vi "Transcriptor LabVIEW to VHDL code Translator Native Functions.vi"(0 "Input":variant=variant("Function Name"=variant(string "Strip Path"), "Input Datatypes"=variant(string[] ["error", "int"]), "Inputs"=variant(string[] ["error in", "x"]), "Node refnum"=variant(refnum<vi> refnum), "Output Datatypes"=variant(string[] ["int"]), "Outputs"=variant(string[] ["a"])), 11 "error in (no error)":errorcluster) -> (4 "Output":variant=variant("Defines"=variant(string[] []), "Includes"=variant(string[] []), "Replaced Code"=variant(string "/* LabVIEW system function 'Strip Path' not found. */")), 15 "error out":errorcluster)   [LabVIEW 2018]
doc: "An example of how to create the Translator to convert the LabVIEW VIs to Arduino C code."
uses:
  <vilib>/regexp/Match Regular Expression.xnode
panel:
  out "Outputs":string[](array[string])
  out "Inputs":string[](array[string])
  out "Output Datatypes":string[](array[string])
  out "Input Datatypes":string[](array[string])
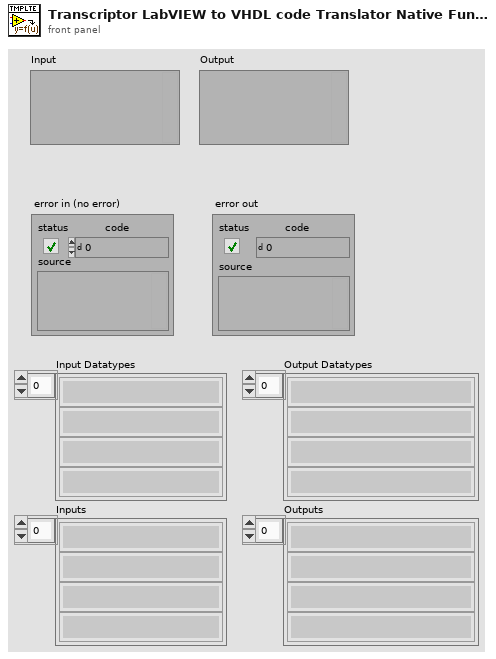
[diagram p1: front panel]
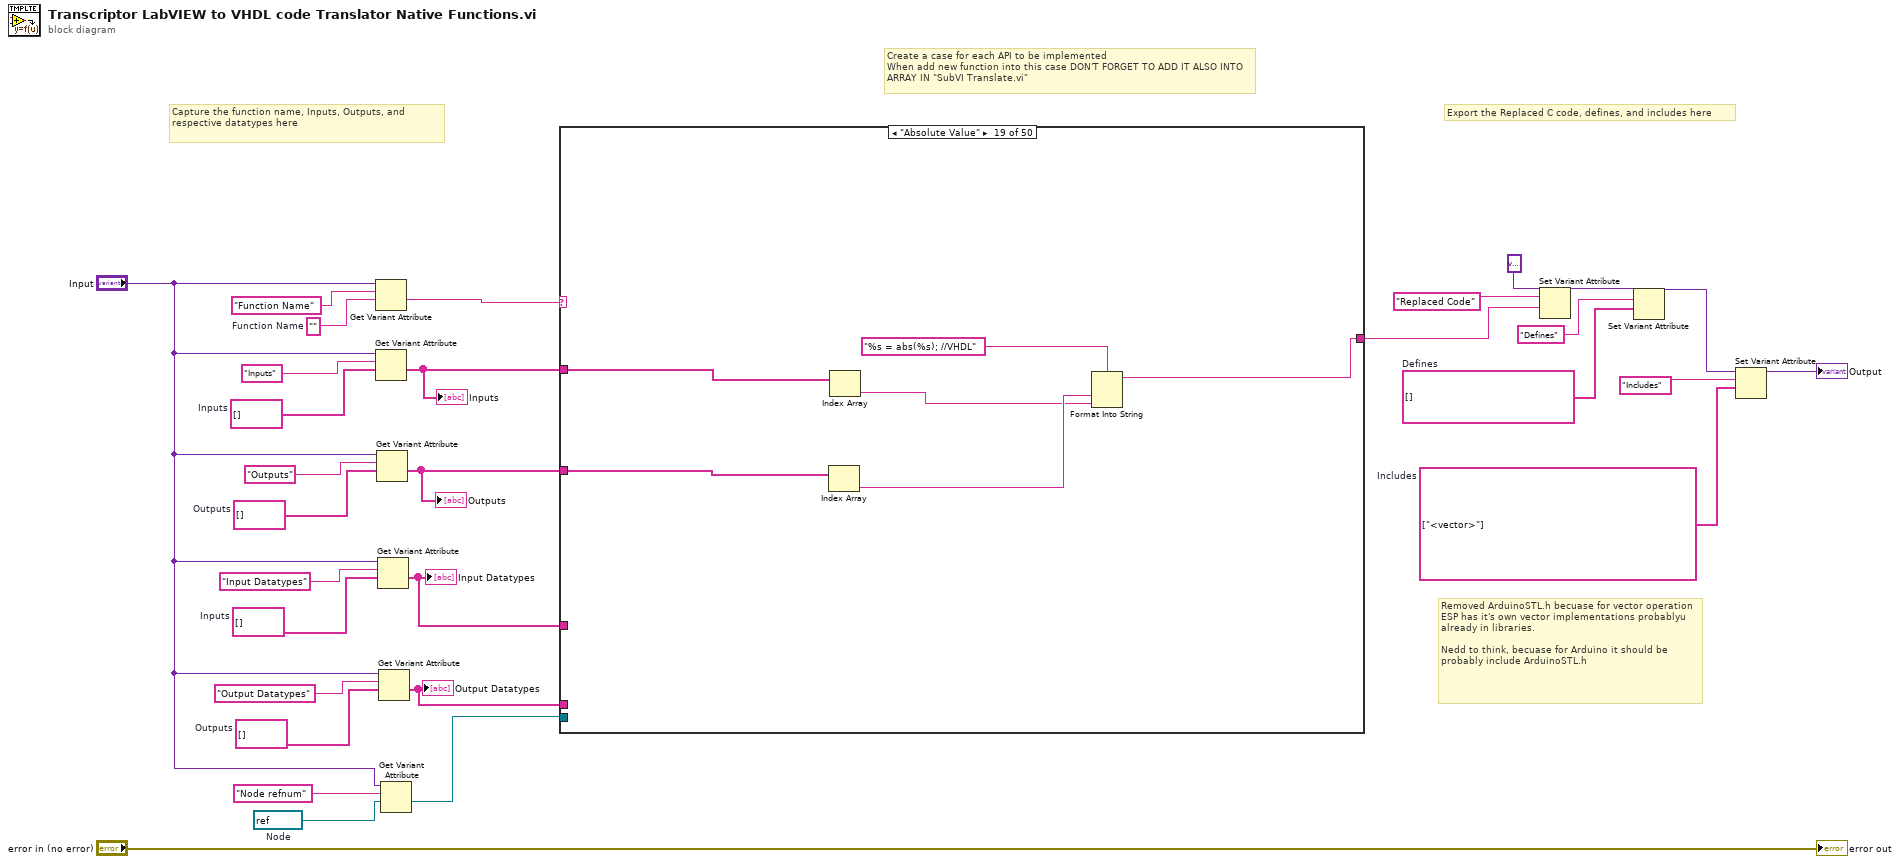
[diagram p0: block diagram]
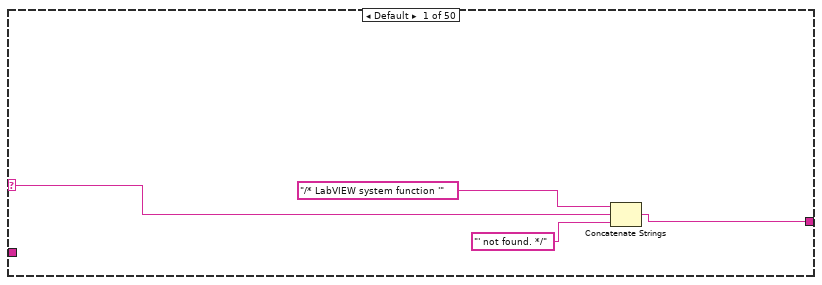
[diagram p2: hidden frame]
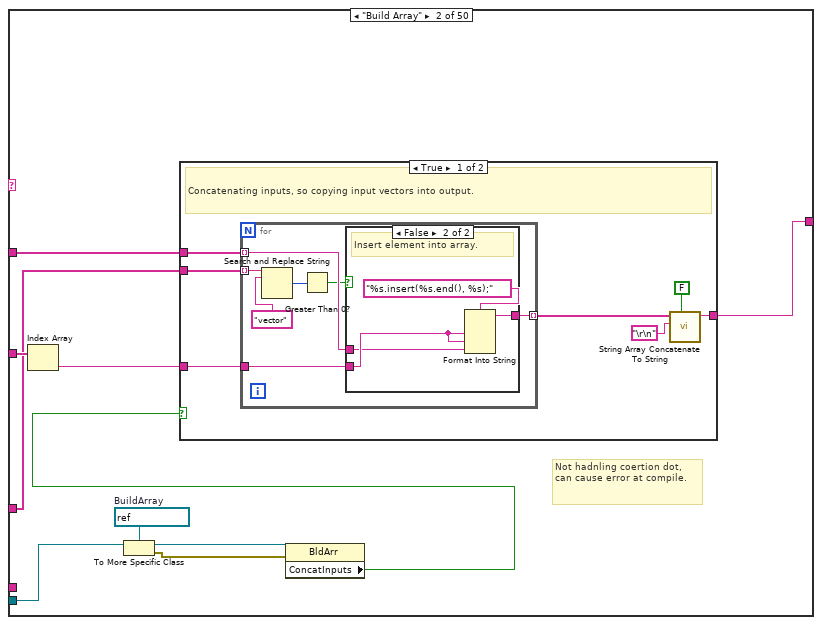
[diagram p3: hidden frame]
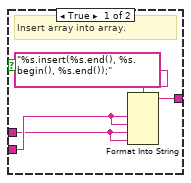
[diagram p4: hidden frame]
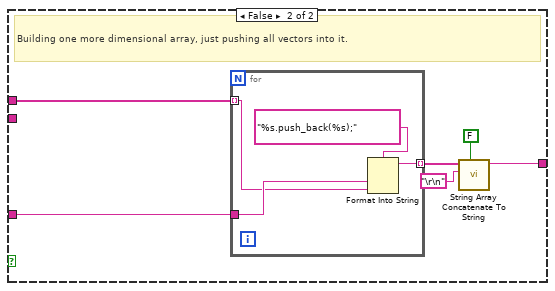
[diagram p5: hidden frame]
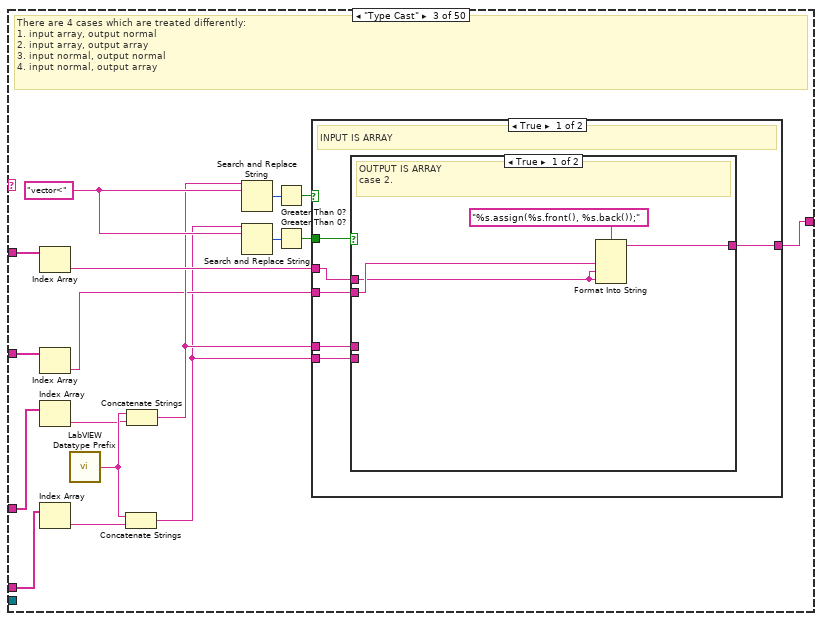
[diagram p6: hidden frame]
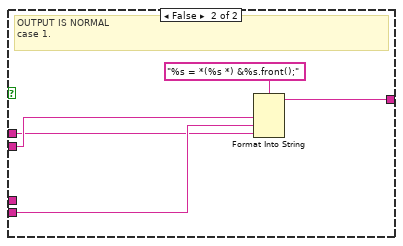
[diagram p7: hidden frame]
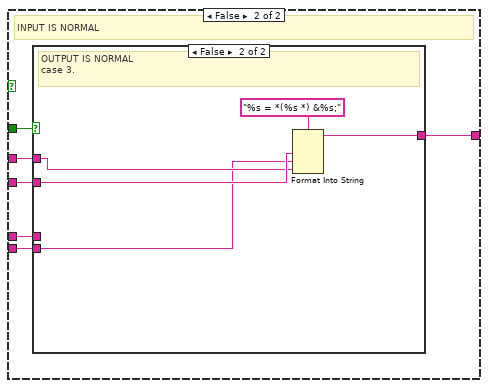
[diagram p8: hidden frame]
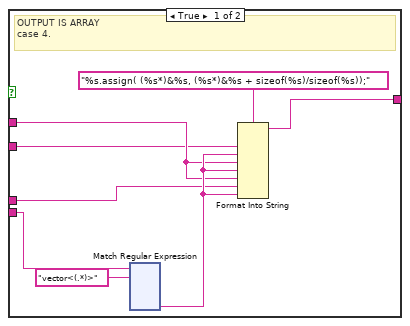
[diagram p9: hidden frame]
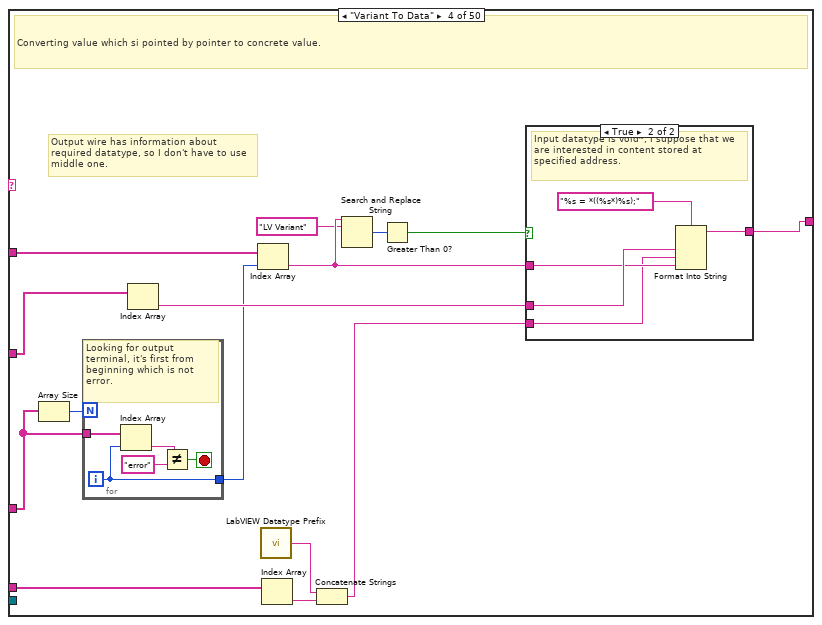
[diagram p10: hidden frame]
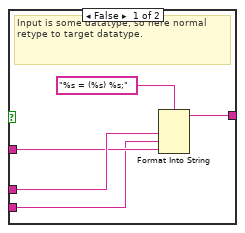
[diagram p11: hidden frame]
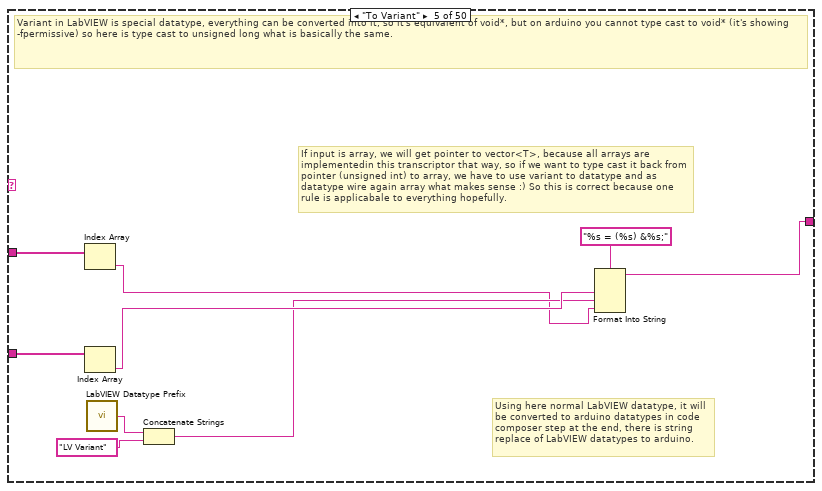
[diagram p12: hidden frame]
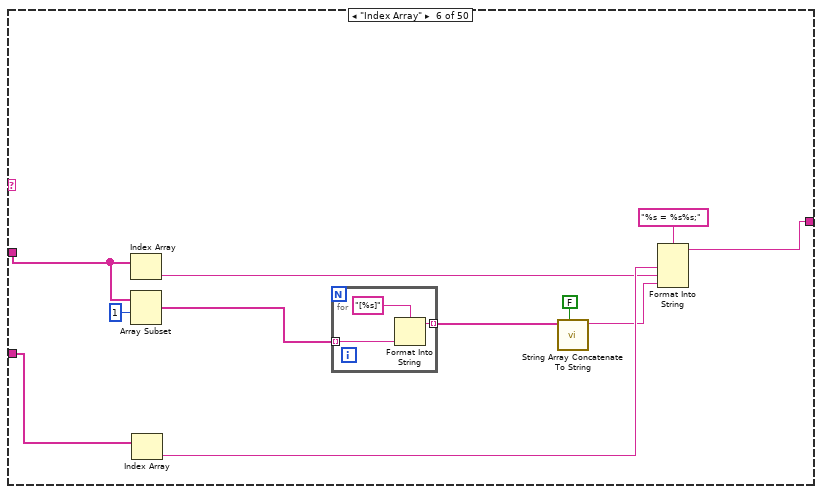
[diagram p13: hidden frame]
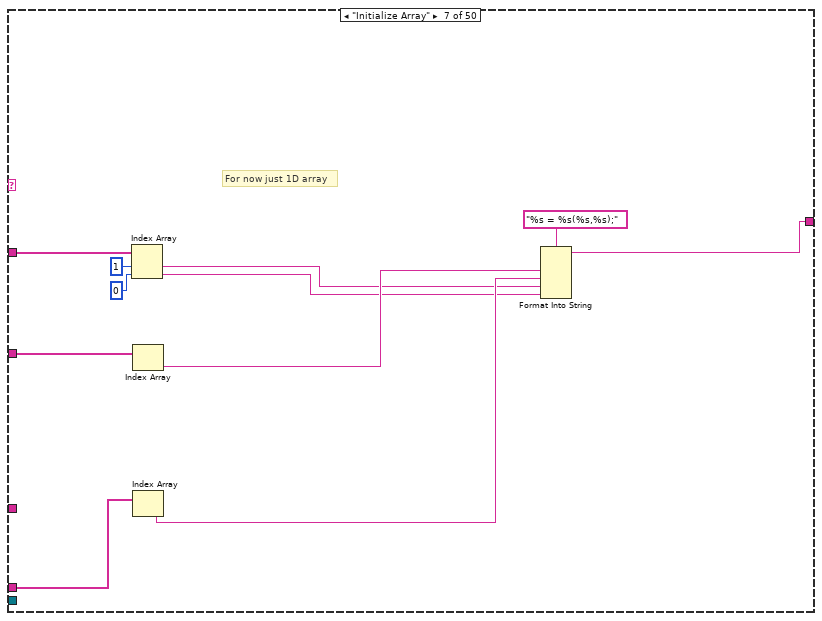
[diagram p14: hidden frame]
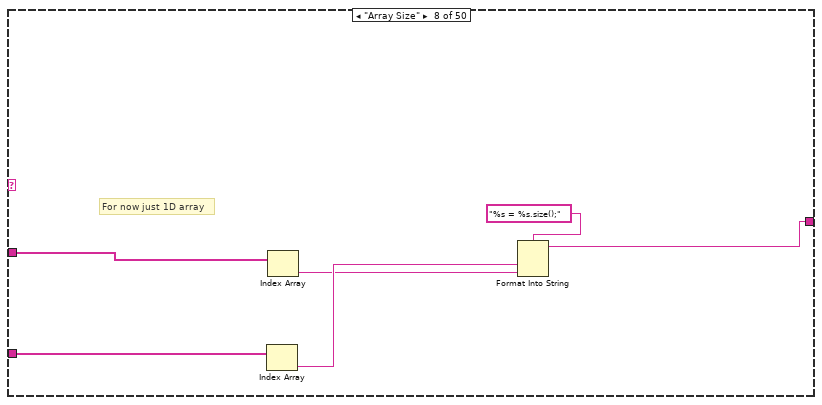
[diagram p15: hidden frame]
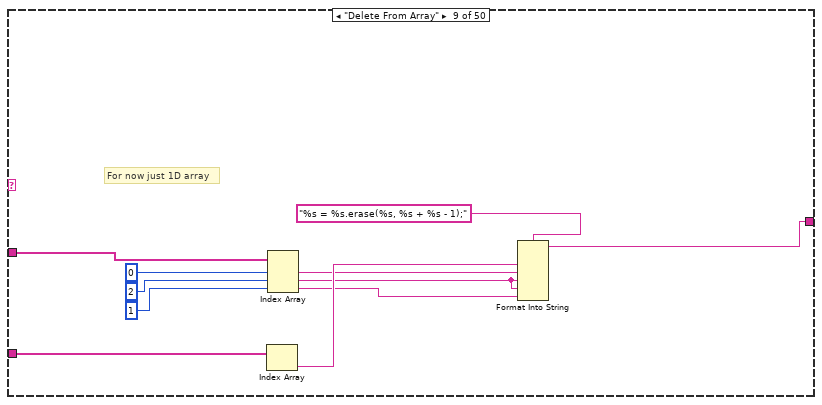
[diagram p16: hidden frame]
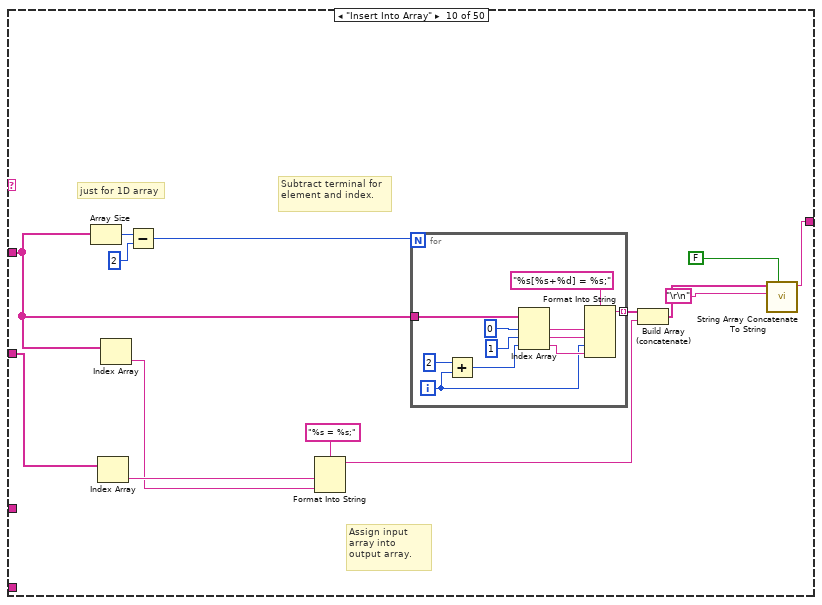
[diagram p17: hidden frame]
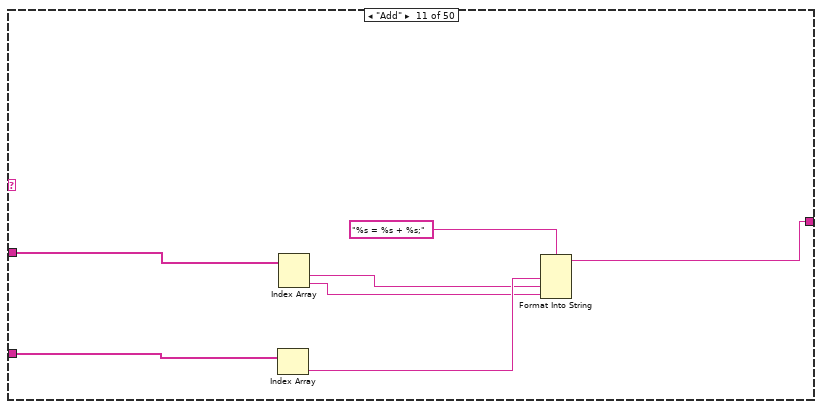
[diagram p18: hidden frame]
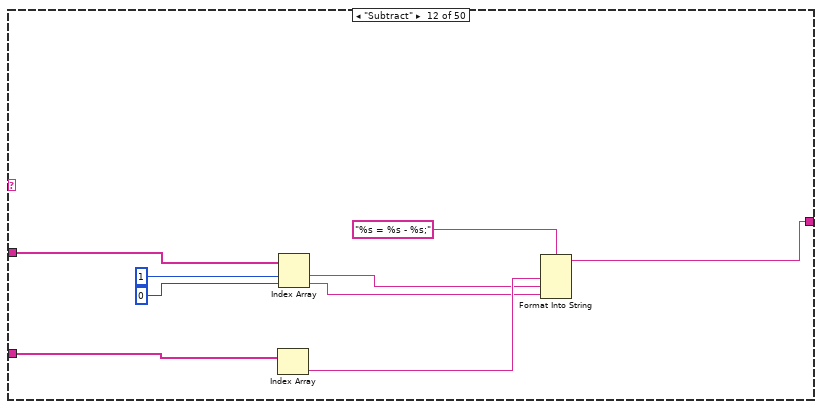
[diagram p19: hidden frame]
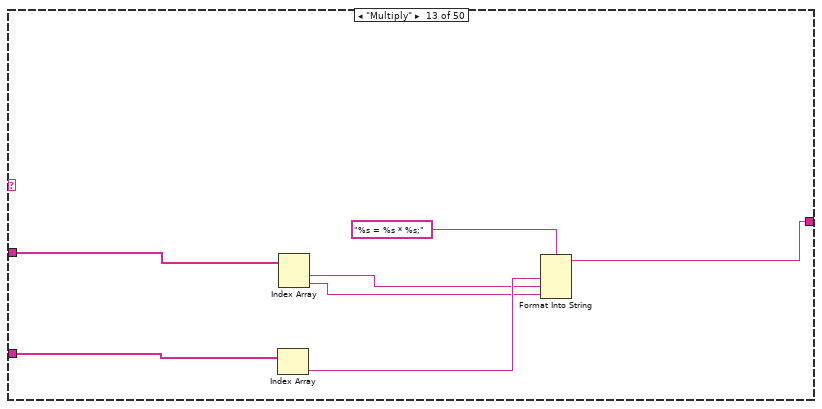
[diagram p20: hidden frame]
diagram:
  w3 = refnum<vi> refnum  # Node
  w7 = string[] []  # Defines
  w15 = string[] []  # Outputs
  w16 = string[] []  # Inputs
  w21 = string[] ["<vector>"]  # Includes
  w26 = string[] []  # Outputs
  w27 = string[] []  # Inputs
  w28 = ""  # Function Name
  # "Removed ArduinoSTL.h becuase for vector operation ESP has it's own vector implementations probablyu already in libraries.\n\nNedd to think, becuase for Arduino it should be probably include ArduinoSTL.h"
  # "Capture the function name, Inputs, Outputs, and respective datatypes here"
  # "Export the Replaced C code, defines, and includes here"
  # "Create a case for each API to be implemented\nWhen add new function into this case DON'T FORGET TO ADD IT ALSO INTO ARRAY IN \"SubVI Translate.vi\""
  n1 = Get Variant Attribute(Variant="Input", name="Function Name", default value (empty Variant)=w28) -> (value=w23:string)  [unwired: 1 in, 3 out]
  n2 = Get Variant Attribute(Variant="Input", name="Inputs", default value (empty Variant)=w27) -> (value=w12:string[])  [unwired: 1 in, 3 out]
  "Inputs" <- w12
  n3 = Get Variant Attribute(Variant="Input", name="Outputs", default value (empty Variant)=w26) -> (value=w13:string[])  [unwired: 1 in, 3 out]
  "Outputs" <- w13
  n4 = Get Variant Attribute(Variant="Input", name="Input Datatypes", default value (empty Variant)=w16) -> (value=w6:string[])  [unwired: 1 in, 3 out]
  "Input Datatypes" <- w6
  n5 = Get Variant Attribute(Variant="Input", name="Output Datatypes", default value (empty Variant)=w15) -> (value=w1:string[])  [unwired: 1 in, 3 out]
  "Output Datatypes" <- w1
  n6 = Get Variant Attribute(Variant="Input", name="Node refnum", default value (empty Variant)=w3) -> (value=w2:refnum<vi>)  [unwired: 1 in, 3 out]
  n7 = case shown="\"Absolute Value\"" w23 {
    selector: w23 -> [w33 _ _ _ _ _ _ _ _ _ _ _ _ _ _ _ _ _ _ _ _ _ _ _ _ _ _ _ _ _ _ _ _ _ _ _ _ _ _ _ _ _ _ _ _ _ _ _ _ _]
    tunnel: [w31 w41 w93 w258 w282 w289 w297 w308 w319 w336 w350 w359 w366 w375 w382 w391 w400 w407 w413 w419 w425 w431 w437 w443 w449 w455 w466 w477 w483 w490 w496 w503 w515 w521 w525 w532 w537 w552 w569 w579 w589 w599 w605 w611 w617 w623 w629 w635 w641 w647] -> w22
    tunnel: w12 -> [_ w43 w92 w251 w281 w288 w307 w313 w324 w329 w356 w365 w372 w381 w388 w397 w406 w412 w418 w424 w430 w436 w442 w448 w454 w460 w465 w474 w489 w495 w502 w509 w512 w524 w528 w534 w536 w554 w566 w576 w586 w598 w604 w610 w616 w622 w628 w634 w640 w646]
    tunnel: w13 -> [_ w44 w91 w257 w280 w293 w306 w311 w322 w332 w354 w363 w370 w379 w386 w395 w404 w410 w416 w422 w428 w434 w440 w446 w452 w458 w470 w481 w487 w493 w500 w507 w519 _ _ w530 w535 w553 w563 w573 w583 w594 w603 w609 w615 w621 w627 w633 w639 w645]
    tunnel: w6 -> [_ w35 w83 w249 _ _ _ _ _ _ _ _ _ _ _ _ _ _ _ _ _ _ _ _ _ _ _ _ _ _ _ _ _ _ _ _ _ _ _ _ _ _ _ _ _ _ _ _ _ _]
    tunnel: w2 -> [_ w40 _ _ _ _ _ _ _ _ _ _ _ _ _ _ _ _ _ _ _ _ _ _ _ _ _ _ _ _ _ _ _ _ _ _ _ _ _ _ _ _ _ _ _ _ _ _ _ _]
    tunnel: w1 -> [_ _ w89 w252 _ _ w302 _ _ _ _ _ _ _ _ _ _ _ _ _ _ _ _ _ _ _ _ _ _ _ _ _ _ _ _ _ _ _ _ _ _ _ _ _ _ _ _ _ _ _]
    frame Default {
      n8 = Concatenate Strings("/* LabVIEW system function '", w33, "' not found. */") -> (w31:string)
    }
    frame "Build Array" {
      w39 = refnum<vi> refnum  # BuildArray
      # "Not hadnling coertion dot, can cause error at compile."
      n9 = Index Array(array=w44) -> (element=w42:string)  [unwired: 1 in]
      n10 = To More Specific Class(target class=w39, reference=w40) -> (specific class reference=w38:refnum<vi>, error out=w37:errorcluster)  [unwired: 1 in]
      n11 = property class="BldArr"(reference=w38, error in=w37) -> ("ConcatInputs"=w36:bool)  [unwired: 2 out]
      n12 = case shown="True" w36 {
        tunnel: w43 -> [w51 w72]
        tunnel: w42 -> [w50 w71]
        tunnel: [w46 w67] -> w41
        tunnel: w35 -> [w45 _]
        frame True {
          # "Concatenating inputs, so copying input vectors into output."
          n13 = for {
            tunnel: w51 -> [w57] mode=indexing
            tunnel: w50 -> [w58]
            tunnel: [w56] -> w49 mode=indexing
            tunnel: w45 -> [w55] mode=indexing
            n14 = Search and Replace String(input string=w55, search string="vector" ("name")) -> (number of replacements=w53:i32)  [unwired: 6 in, 3 out]
            n15 = Greater Than 0?(x=w53) -> (x > 0?=w52:bool)
            n16 = case shown="False" w52 {
              tunnel: w58 -> [w61 w65]
              tunnel: w57 -> [w60 w64]
              tunnel: [w59 w63] -> w56
              frame True {
                # "Insert array into array."
                n17 = Format Into String(format string="%s.insert(%s.end(), %s.begin(), %s.end());" ("name"), w61, w61, w60, w60) -> (resulting string=w59:string)  [unwired: 2 in, 1 out]
              }
              frame False {
                # "Insert element into array."
                n18 = Format Into String(format string="%s.insert(%s.end(), %s);" ("name"), w65, w65, w64) -> (resulting string=w63:string)  [unwired: 2 in, 1 out]
              }
            }
          }
          n19 = call "String Array Concatenate To String.vi"("insert last delimiter?"=FALSE, "Delimiter char"="\r\n", "Array String In"=w49) -> ("String"=w46:string)  [unwired: 8 in]
        }
        frame False {
          # "Building one more dimensional array, just pushing all vectors into it."
          n20 = for {
            tunnel: w72 -> [w74] mode=indexing
            tunnel: w71 -> [w75]
            tunnel: [w73] -> w70 mode=indexing
            n21 = Format Into String(format string="%s.push_back(%s);" ("name"), w75, w74) -> (resulting string=w73:string)  [unwired: 2 in, 1 out]
          }
          n22 = call "String Array Concatenate To String.vi"("insert last delimiter?"=FALSE, "Delimiter char"="\r\n", "Array String In"=w70) -> ("String"=w67:string)  [unwired: 8 in]
        }
      }
    }
    frame "Type Cast" {
      w86 = "vector<" ("search string")
      # "There are 4 cases which are treated differently:\n1. input array, output normal\n2. input array, output array\n3. input normal, output normal\n4. input normal, output array"
      n23 = Index Array(array=w92) -> (element=w82:string)  [unwired: 1 in]
      n24 = Index Array(array=w91) -> (element=w78:string)  [unwired: 1 in]
      n25 = Index Array(array=w83) -> (element=w80:string)  [unwired: 1 in]
      n26 = Index Array(array=w89) -> (element=w90:string)  [unwired: 1 in]
      n27 = call "LabVIEW Datatype Prefix.vi"() -> ("datatype prefix"=w81:string)
      n28 = Concatenate Strings(w81, w90) -> (w77:string)
      n29 = Concatenate Strings(w81, w80) -> (w79:string)
      n30 = Search and Replace String(input string=w79, search string=w86) -> (number of replacements=w88:i32)  [unwired: 6 in, 3 out]
      n31 = Search and Replace String(input string=w77, search string=w86) -> (number of replacements=w87:i32)  [unwired: 6 in, 3 out]
      n32 = Greater Than 0?(x=w88) -> (x > 0?=w85:bool)
      n33 = Greater Than 0?(x=w87) -> (x > 0?=w84:bool)
      n34 = case shown="True" w85 {
        tunnel: [w99 w114] -> w93
        tunnel: w82 -> [w98 w113]
        tunnel: w78 -> [w97 w112]
        tunnel: w84 -> [w96 w111]
        tunnel: w79 -> [w95 w110]
        tunnel: w77 -> [w94 w109]
        frame True {
          # "INPUT IS ARRAY"
          n35 = case shown="True" w96 {
            tunnel: [w102 w107] -> w99
            tunnel: w97 -> [w101 w106]
            tunnel: w98 -> [w100 w104]
            tunnel: w95 -> [_ _]
            tunnel: w94 -> [_ w105]
            frame True {
              # "OUTPUT IS ARRAY\ncase 2."
              n36 = Format Into String(format string="%s.assign(%s.front(), %s.back());" ("name"), w101, w100, w100) -> (resulting string=w102:string)  [unwired: 2 in, 1 out]
            }
            frame False {
              # "OUTPUT IS NORMAL\ncase 1."
              n37 = Format Into String(format string="%s = *(%s *) &%s.front();" ("name"), w106, w105, w104) -> (resulting string=w107:string)  [unwired: 2 in, 1 out]
            }
          }
        }
        frame False {
          # "INPUT IS NORMAL"
          n38 = case shown="False" w111 {
            tunnel: [w119 w242] -> w114
            tunnel: w112 -> [w117 w241]
            tunnel: w113 -> [w118 w240]
            tunnel: w110 -> [w116 _]
            tunnel: w109 -> [w115 w239]
            frame True {
              # "OUTPUT IS ARRAY\ncase 4."
              n39 = xnode "Match Regular Expression"("input string"=w115, "regular expression"="vector<(.*)>") -> ("submatch 1"=w120:string)  [unwired: 4 in, 5 out]
              n40 = Format Into String(format string="%s.assign( (%s*)&%s, (%s*)&%s + sizeof(%s)/sizeof(%s));" ("name"), w117, w120, w118, w120, w118, w116, w120) -> (resulting string=w119:string)  [unwired: 2 in, 1 out]
            }
            frame False {
              # "OUTPUT IS NORMAL\ncase 3."
              n41 = Format Into String(format string="%s = *(%s *) &%s;" ("name"), w241, w239, w240) -> (resulting string=w242:string)  [unwired: 2 in, 1 out]
            }
          }
        }
      }
    }
    frame "Variant To Data" {
      # "Output wire has information about required datatype, so I don't have to use middle one."
      # "Converting value which si pointed by pointer to concrete value."
      n42 = Array Size(array=w249) -> (size(s)=w250:i32)
      n43 = for {
        N: w250 -> [_]
        tunnel: w249 -> [w273]
        tunnel: [w269] -> w248
        i -> [w269]
        stop <- w272 stop-if-true
        # "Looking for output terminal, it's first from beginning which is not error."
        n44 = Index Array(array=w273, index=w269) -> (element=w271:string)
        n45 = Not Equal?(x=w271, y="error") -> (x != y?=w272:bool)
      }
      n46 = Index Array(array=w257) -> (element=w256:string)  [unwired: 1 in]
      n47 = Index Array(array=w251, index=w248) -> (element=w247:string)
      n48 = call "LabVIEW Datatype Prefix.vi"() -> ("datatype prefix"=w253:string)
      n49 = Index Array(array=w252) -> (element=w255:string)  [unwired: 1 in]
      n50 = Concatenate Strings(w253, w255) -> (w254:string)
      n51 = Search and Replace String(input string=w247, search string="LV Variant") -> (number of replacements=w245:i32)  [unwired: 6 in, 3 out]
      n52 = Greater Than 0?(x=w245) -> (x > 0?=w244:bool)
      n53 = case shown="True" w244 {
        tunnel: [w262 w267] -> w258
        tunnel: w256 -> [w261 w266]
        tunnel: w247 -> [w260 w265]
        tunnel: w254 -> [w259 w264]
        frame False {
          # "Input is some datatype, so here normal retype to target datatype."
          n54 = Format Into String(format string="%s = (%s) %s;" ("name"), w261, w259, w260) -> (resulting string=w262:string)  [unwired: 2 in, 1 out]
        }
        frame True {
          # "Input datatype is void*, I suppose that we are interested in content stored at specified address."
          n55 = Format Into String(format string="%s = *((%s*)%s);" ("name"), w266, w264, w265) -> (resulting string=w267:string)  [unwired: 2 in, 1 out]
        }
      }
    }
    frame "To Variant" {
      # "If input is array, we will get pointer to vector<T>, because all arrays are implementedin this transcriptor that way, so if we want to type cast it back from pointer (unsigned int) to array, we have to use variant to datatype and as datatype wire again array what makes sense :) So this is correct because one rule is applicabale to everything hopefully."
      # "Using here normal LabVIEW datatype, it will be converted to arduino datatypes in code composer step at the end, there is string replace of LabVIEW datatypes to arduino."
      # "Variant in LabVIEW is special datatype, everything can be converted into it, so it's equivalent of void*, but on arduino you cannot type cast to void* (it's showing -fpermissive) so here is type cast to unsigned long what is basically the same."
      n56 = Index Array(array=w281) -> (element=w275:string)  [unwired: 1 in]
      n57 = Index Array(array=w280) -> (element=w279:string)  [unwired: 1 in]
      n58 = call "LabVIEW Datatype Prefix.vi"() -> ("datatype prefix"=w278:string)
      n59 = Concatenate Strings(w278, "LV Variant" ("string")) -> (w276:string)
      n60 = Format Into String(format string="%s = (%s) &%s;", w279, w276, w275) -> (resulting string=w282:string)  [unwired: 2 in, 1 out]
    }
    frame "Index Array" {
      n61 = Index Array(array=w288) -> (element=w290:string)  [unwired: 1 in]
      n62 = Array Subset(array=w288, index=1) -> (w286:string[])  [unwired: 1 in]
      n63 = Index Array(array=w293) -> (element=w291:string)  [unwired: 1 in]
      n64 = for {
        tunnel: w286 -> [w295] mode=indexing
        tunnel: [w294] -> w284 mode=indexing
        n65 = Format Into String(format string="[%s]", w295) -> (resulting string=w294:string)  [unwired: 2 in, 1 out]
      }
      n66 = call "String Array Concatenate To String.vi"("insert last delimiter?"=FALSE, "Array String In"=w284) -> ("String"=w283:string)  [unwired: 9 in]
      n67 = Format Into String(format string="%s = %s%s;", w291, w290, w283) -> (resulting string=w289:string)  [unwired: 2 in, 1 out]
    }
    frame "Initialize Array" {
      # "For now just 1D array"
      n68 = Index Array(array=w307, index #1=1 ("index"), index #2=0 ("index")) -> (element #1=w299:string, element #2=w298:string)
      n69 = Index Array(array=w306) -> (element=w304:string)  [unwired: 1 in]
      n70 = Index Array(array=w302) -> (element=w303:string)  [unwired: 1 in]
      n71 = Format Into String(format string="%s = %s(%s,%s);", w304, w303, w299, w298) -> (resulting string=w297:string)  [unwired: 2 in, 1 out]
    }
    frame "Array Size" {
      # "For now just 1D array"
      n72 = Index Array(array=w311) -> (element=w310:string)  [unwired: 1 in]
      n73 = Index Array(array=w313) -> (element=w309:string)  [unwired: 1 in]
      n74 = Format Into String(format string="%s = %s.size();", w310, w309) -> (resulting string=w308:string)  [unwired: 2 in, 1 out]
    }
    frame "Delete From Array" {
      # "For now just 1D array"
      n75 = Index Array(array=w322) -> (element=w321:string)  [unwired: 1 in]
      n76 = Index Array(array=w324, index #1=0 ("index"), index #2=2 ("index"), index #3=1 ("index")) -> (element #1=w320:string, element #2=w315:string, element #3=w314:string)
      n77 = Format Into String(format string="%s = %s.erase(%s, %s + %s - 1);", w321, w320, w315, w315, w314) -> (resulting string=w319:string)  [unwired: 2 in, 1 out]
    }
    frame "Insert Into Array" {
      # "just for 1D array"
      # "Subtract terminal for element and index."
      # "Assign input array into output array."
      n78 = Array Size(array=w329) -> (size(s)=w334:i32)
      n79 = Index Array(array=w332) -> (element=w330:string)  [unwired: 1 in]
      n80 = Index Array(array=w329) -> (element=w328:string)  [unwired: 1 in]
      n81 = Subtract(x=w334, y=2) -> (x-y=w335:i32)
      n82 = Format Into String(format string="%s = %s;", w330, w328) -> (resulting string=w326:string)  [unwired: 2 in, 1 out]
      n83 = for {
        N: w335 -> [_]
        tunnel: w329 -> [w346]
        tunnel: [w347] -> w327 mode=indexing
        i -> [w342]
        n84 = Add(x=2, y=w342) -> (x+y=w341:i32)
        n85 = Index Array(array=w346, index #1=0 ("index"), index #2=1 ("index"), index #3=w341) -> (element #1=w339:string, element #2=w348:string, element #3=w344:string)
        n86 = Format Into String(format string="%s[%s+%d] = %s;", w339, w348, w342, w344) -> (resulting string=w347:string)  [unwired: 2 in, 1 out]
      }
      n87 = Build Array (concatenate)(w327, w326) -> (w325:string[])
      n88 = call "String Array Concatenate To String.vi"("insert last delimiter?"=FALSE, "Delimiter char"="\r\n", "Array String In"=w325) -> ("String"=w336:string)  [unwired: 8 in]
    }
    frame "Add" {
      n89 = Index Array(array=w354) -> (element=w353:string)  [unwired: 1 in]
      n90 = Index Array(array=w356) -> (element #1=w352:string, element #2=w351:string)  [unwired: 2 in]
      n91 = Format Into String(format string="%s = %s + %s;", w353, w352, w351) -> (resulting string=w350:string)  [unwired: 2 in, 1 out]
    }
    frame "Subtract" {
      n92 = Index Array(array=w363) -> (element=w362:string)  [unwired: 1 in]
      n93 = Index Array(array=w365, index #1=1 ("index"), index #2=0 ("index")) -> (element #1=w361:string, element #2=w360:string)
      n94 = Format Into String(format string="%s = %s - %s;", w362, w361, w360) -> (resulting string=w359:string)  [unwired: 2 in, 1 out]
    }
    frame "Multiply" {
      n95 = Index Array(array=w370) -> (element=w369:string)  [unwired: 1 in]
      n96 = Index Array(array=w372) -> (element #1=w368:string, element #2=w367:string)  [unwired: 2 in]
      n97 = Format Into String(format string="%s = %s * %s;", w369, w368, w367) -> (resulting string=w366:string)  [unwired: 2 in, 1 out]
    }
    frame "Divide" {
      n98 = Index Array(array=w379) -> (element=w378:string)  [unwired: 1 in]
      n99 = Index Array(array=w381, index #1=1 ("index"), index #2=0 ("index")) -> (element #1=w377:string, element #2=w376:string)
      n100 = Format Into String(format string="%s = %s / %s;", w378, w377, w376) -> (resulting string=w375:string)  [unwired: 2 in, 1 out]
    }
    frame "Equal?" {
      n101 = Index Array(array=w386) -> (element=w385:string)  [unwired: 1 in]
      n102 = Index Array(array=w388) -> (element #1=w384:string, element #2=w383:string)  [unwired: 2 in]
      n103 = Format Into String(format string="%s = %s == %s;", w385, w384, w383) -> (resulting string=w382:string)  [unwired: 2 in, 1 out]
    }
    frame "Less?" {
      n104 = Index Array(array=w395) -> (element=w394:string)  [unwired: 1 in]
      n105 = Index Array(array=w397, index #1=1 ("index"), index #2=0 ("index")) -> (element #1=w393:string, element #2=w392:string)
      n106 = Format Into String(format string="%s = %s < %s;", w394, w393, w392) -> (resulting string=w391:string)  [unwired: 2 in, 1 out]
    }
    frame "Greater?" {
      n107 = Index Array(array=w404) -> (element=w403:string)  [unwired: 1 in]
      n108 = Index Array(array=w406, index #1=1 ("index"), index #2=0 ("index")) -> (element #1=w402:string, element #2=w401:string)
      n109 = Format Into String(format string="%s = %s > %s;", w403, w402, w401) -> (resulting string=w400:string)  [unwired: 2 in, 1 out]
    }
    frame "Not" {
      n110 = Index Array(array=w410) -> (element=w409:string)  [unwired: 1 in]
      n111 = Index Array(array=w412) -> (element=w408:string)  [unwired: 1 in]
      n112 = Format Into String(format string="%s = !%s;", w409, w408) -> (resulting string=w407:string)  [unwired: 2 in, 1 out]
    }
    frame "Absolute Value" {
      n113 = Index Array(array=w416) -> (element=w415:string)  [unwired: 1 in]
      n114 = Index Array(array=w418) -> (element=w414:string)  [unwired: 1 in]
      n115 = Format Into String(format string="%s = abs(%s); //VHDL", w415, w414) -> (resulting string=w413:string)  [unwired: 2 in, 1 out]
    }
    frame "Increment" {
      n116 = Index Array(array=w422) -> (element=w421:string)  [unwired: 1 in]
      n117 = Index Array(array=w424) -> (element=w420:string)  [unwired: 1 in]
      n118 = Format Into String(format string="%s = %s + 1;", w421, w420) -> (resulting string=w419:string)  [unwired: 2 in, 1 out]
    }
    frame "Decrement" {
      n119 = Index Array(array=w428) -> (element=w427:string)  [unwired: 1 in]
      n120 = Index Array(array=w430) -> (element=w426:string)  [unwired: 1 in]
      n121 = Format Into String(format string="%s = %s - 1;", w427, w426) -> (resulting string=w425:string)  [unwired: 2 in, 1 out]
    }
    frame "Equal To 0?" {
      n122 = Index Array(array=w434) -> (element=w433:string)  [unwired: 1 in]
      n123 = Index Array(array=w436) -> (element=w432:string)  [unwired: 1 in]
      n124 = Format Into String(format string="%s = (%s == 0);", w433, w432) -> (resulting string=w431:string)  [unwired: 2 in, 1 out]
    }
    frame "Greater Than 0?" {
      n125 = Index Array(array=w440) -> (element=w439:string)  [unwired: 1 in]
      n126 = Index Array(array=w442) -> (element=w438:string)  [unwired: 1 in]
      n127 = Format Into String(format string="%s = (%s > 0);", w439, w438) -> (resulting string=w437:string)  [unwired: 2 in, 1 out]
    }
    frame "Less Than 0?" {
      n128 = Index Array(array=w446) -> (element=w445:string)  [unwired: 1 in]
      n129 = Index Array(array=w448) -> (element=w444:string)  [unwired: 1 in]
      n130 = Format Into String(format string="%s = (%s < 0);", w445, w444) -> (resulting string=w443:string)  [unwired: 2 in, 1 out]
    }
    frame "Greater Or Equal To 0?" {
      n131 = Index Array(array=w452) -> (element=w451:string)  [unwired: 1 in]
      n132 = Index Array(array=w454) -> (element=w450:string)  [unwired: 1 in]
      n133 = Format Into String(format string="%s = (%s >= 0);", w451, w450) -> (resulting string=w449:string)  [unwired: 2 in, 1 out]
    }
    frame "Less Or Equal To 0?" {
      n134 = Index Array(array=w458) -> (element=w457:string)  [unwired: 1 in]
      n135 = Index Array(array=w460) -> (element=w456:string)  [unwired: 1 in]
      n136 = Format Into String(format string="%s = (%s <= 0);", w457, w456) -> (resulting string=w455:string)  [unwired: 2 in, 1 out]
    }
    frame "Greater Or Equal?" {
      n137 = Array Size(array=w465) -> (size(s)=w463:i32)
      n138 = Decrement(x=w463) -> (x-1=w461:i32)
      n139 = Decrement(x=w463) -> (x-1=w464:i32)
      n140 = Decrement(x=w461) -> (x-1=w462:i32)
      n141 = Index Array(array=w470) -> (element=w469:string)  [unwired: 1 in]
      n142 = Index Array(array=w465, index #1=w464, index #2=w462) -> (element #1=w468:string, element #2=w467:string)
      n143 = Format Into String(format string="%s = (%s >= %s);", w469, w468, w467) -> (resulting string=w466:string)  [unwired: 2 in, 1 out]
    }
    frame "Less Or Equal?" {
      n144 = Array Size(array=w474) -> (size(s)=w476:i32)
      n145 = Decrement(x=w476) -> (x-1=w475:i32)
      n146 = Decrement(x=w476) -> (x-1=w473:i32)
      n147 = Decrement(x=w475) -> (x-1=w472:i32)
      n148 = Index Array(array=w481) -> (element=w480:string)  [unwired: 1 in]
      n149 = Index Array(array=w474, index #1=w473, index #2=w472) -> (element #1=w479:string, element #2=w478:string)
      n150 = Format Into String(format string="%s = (%s <= %s);", w480, w479, w478) -> (resulting string=w477:string)  [unwired: 2 in, 1 out]
    }
    frame "Not Equal?" {
      n151 = Index Array(array=w487) -> (element=w486:string)  [unwired: 1 in]
      n152 = Index Array(array=w489) -> (element #1=w485:string, element #2=w484:string)  [unwired: 2 in]
      n153 = Format Into String(format string="%s = (%s != %s);", w486, w485, w484) -> (resulting string=w483:string)  [unwired: 2 in, 1 out]
    }
    frame "Not Equal To 0?" {
      n154 = Index Array(array=w493) -> (element=w492:string)  [unwired: 1 in]
      n155 = Index Array(array=w495) -> (element=w491:string)  [unwired: 1 in]
      n156 = Format Into String(format string="%s = (%s != 0);", w492, w491) -> (resulting string=w490:string)  [unwired: 2 in, 1 out]
    }
    frame "And" {
      n157 = Index Array(array=w500) -> (element=w499:string)  [unwired: 1 in]
      n158 = Index Array(array=w502) -> (element #1=w498:string, element #2=w497:string)  [unwired: 2 in]
      n159 = Format Into String(format string="%s = %s && %s;", w499, w498, w497) -> (resulting string=w496:string)  [unwired: 2 in, 1 out]
    }
    frame "Or" {
      n160 = Index Array(array=w507) -> (element=w506:string)  [unwired: 1 in]
      n161 = Index Array(array=w509) -> (element #1=w505:string, element #2=w504:string)  [unwired: 2 in]
      n162 = Format Into String(format string="%s = %s || %s;", w506, w505, w504) -> (resulting string=w503:string)  [unwired: 2 in, 1 out]
    }
    frame "Exclusive Or" {
      n163 = Array Size(array=w512) -> (size(s)=w514:i32)
      n164 = Decrement(x=w514) -> (x-1=w513:i32)
      n165 = Decrement(x=w514) -> (x-1=w511:i32)
      n166 = Decrement(x=w513) -> (x-1=w510:i32)
      n167 = Index Array(array=w519) -> (element=w518:string)  [unwired: 1 in]
      n168 = Index Array(array=w512, index #1=w511, index #2=w510) -> (element #1=w517:string, element #2=w516:string)
      n169 = Format Into String(format string="%s = %s ^ %s;", w518, w517, w516) -> (resulting string=w515:string)  [unwired: 2 in, 1 out]
    }
    frame "To Lower Case" {
      n170 = Index Array(array=w524) -> (element=w522:string)  [unwired: 1 in]
      n171 = Format Into String(format string="%s.toLowerCase();", w522) -> (resulting string=w521:string)  [unwired: 2 in, 1 out]
    }
    frame "To Upper Case" {
      n172 = Index Array(array=w528) -> (element=w526:string)  [unwired: 1 in]
      n173 = Format Into String(format string="%s.toUpperCase();", w526) -> (resulting string=w525:string)  [unwired: 2 in, 1 out]
    }
    frame "String Length" {
      n174 = Index Array(array=w530) -> (element=w529:string)  [unwired: 1 in]
      n175 = Index Array(array=w534) -> (element=w531:string)  [unwired: 1 in]
      n176 = Format Into String(format string="%s = %s.length();", w529, w531) -> (resulting string=w532:string)  [unwired: 2 in, 1 out]
    }
    frame "String Subset" {
      # "If more output wired take one with highes index.\n\nI'm interested just in index, no string outputs."
      n177 = Array Size(array=w535) -> (size(s)=w541:i32)
      n178 = Greater?(x=w541, y=1) -> (0:w542:bool)
      n179 = Index Array(array=w536, index #1=2 ("index"), index #2=1 ("index"), index #3=0 ("index")) -> (element #1=w548:string, element #2=w547:string, element #3=w545:string)
      n180 = Decrement(x=w541) -> (x-1=w539:i32)
      n181 = Select(t=w539, s=w542, f=0) -> (s? t:f=w538:i32)
      n182 = Index Array(array=w535, index=w538) -> (element=w549:string)
      n183 = Format Into String(format string="%s = %s.substring(%s,%s);", w549, w548, w547, w545) -> (resulting string=w537:string)  [unwired: 2 in, 1 out]
    }
    frame "Match Pattern" {
      n184 = Index Array(array=w554, index #1=1 ("index"), index #2=0 ("index"), index #3=2 ("index")) -> (element #1=w558:string, element #2=w559:string, element #3=w561:string)
      n185 = Index Array(array=w553) -> (element=w557:string)  [unwired: 1 in]
      n186 = Format Into String(format string="%s = %s.indexOf(%s,%s);", w557, w558, w559, w561) -> (resulting string=w552:string)  [unwired: 2 in, 1 out]
    }
    frame "Decimal String To Number" {
      # "Here we are hoping that user wired just one input and just one output."
      n187 = Array Size(array=w566) -> (size(s)=w568:i32)
      n188 = Array Size(array=w563) -> (size(s)=w565:i32)
      n189 = Decrement(x=w568) -> (x-1=w567:i32)
      n190 = Decrement(x=w565) -> (x-1=w564:i32)
      n191 = Index Array(array=w566, index=w567) -> (element=w572:string)
      n192 = Index Array(array=w563, index=w564) -> (element=w571:string)
      n193 = Format Into String(format string="%s = %s.toInt();", w571, w572) -> (resulting string=w569:string)  [unwired: 2 in, 1 out]
    }
    frame "Number To Fractional String" {
      # "NOT IMPLEMENTED PRECISION TERMINAL!"
      # "Here we are hoping that user wired just one input and just one output."
      n194 = Array Size(array=w576) -> (size(s)=w578:i32)
      n195 = Array Size(array=w573) -> (size(s)=w575:i32)
      n196 = Decrement(x=w578) -> (x-1=w577:i32)
      n197 = Decrement(x=w575) -> (x-1=w574:i32)
      n198 = Index Array(array=w576, index=w577) -> (element=w582:string)
      n199 = Index Array(array=w573, index=w574) -> (element=w581:string)
      n200 = Format Into String(format string="%s = String(%s);", w581, w582) -> (resulting string=w579:string)  [unwired: 2 in, 1 out]
    }
    frame "Fract/Exp String To Number" {
      # "Here we are hoping that user wired just one input and just one output."
      n201 = Array Size(array=w586) -> (size(s)=w588:i32)
      n202 = Array Size(array=w583) -> (size(s)=w585:i32)
      n203 = Decrement(x=w588) -> (x-1=w587:i32)
      n204 = Decrement(x=w585) -> (x-1=w584:i32)
      n205 = Index Array(array=w586, index=w587) -> (element=w592:string)
      n206 = Index Array(array=w583, index=w584) -> (element=w591:string)
      n207 = Format Into String(format string="%s = %s.toFloat();", w591, w592) -> (resulting string=w589:string)  [unwired: 2 in, 1 out]
    }
    frame "Number To Decimal String" {
      # "Here we are hoping that user wired just one input and just one output."
      n208 = Array Size(array=w598) -> (size(s)=w597:i32)
      n209 = Array Size(array=w594) -> (size(s)=w595:i32)
      n210 = Decrement(x=w597) -> (x-1=w596:i32)
      n211 = Decrement(x=w595) -> (x-1=w593:i32)
      n212 = Index Array(array=w598, index=w596) -> (element=w602:string)
      n213 = Index Array(array=w594, index=w593) -> (element=w601:string)
      n214 = Format Into String(format string="%s = String(%s);", w601, w602) -> (resulting string=w599:string)  [unwired: 2 in, 1 out]
    }
    frame "To Unsigned Long Integer" {
      n215 = Index Array(array=w604) -> (element=w608:string)  [unwired: 1 in]
      n216 = Index Array(array=w603) -> (element=w607:string)  [unwired: 1 in]
      n217 = Format Into String(format string="%s = (unsigned long) %s;", w607, w608) -> (resulting string=w605:string)  [unwired: 2 in, 1 out]
    }
    frame "To Double Precision Float" {
      n218 = Index Array(array=w610) -> (element=w614:string)  [unwired: 1 in]
      n219 = Index Array(array=w609) -> (element=w613:string)  [unwired: 1 in]
      n220 = Format Into String(format string="%s = (double) %s;", w613, w614) -> (resulting string=w611:string)  [unwired: 2 in, 1 out]
    }
    frame "To Single Precision Float" {
      n221 = Index Array(array=w616) -> (element=w620:string)  [unwired: 1 in]
      n222 = Index Array(array=w615) -> (element=w619:string)  [unwired: 1 in]
      n223 = Format Into String(format string="%s = (float) %s;", w619, w620) -> (resulting string=w617:string)  [unwired: 2 in, 1 out]
    }
    frame "To Unsigned Word Integer" {
      n224 = Index Array(array=w622) -> (element=w626:string)  [unwired: 1 in]
      n225 = Index Array(array=w621) -> (element=w625:string)  [unwired: 1 in]
      n226 = Format Into String(format string="%s = (unsigned short) %s;", w625, w626) -> (resulting string=w623:string)  [unwired: 2 in, 1 out]
    }
    frame "To Unsigned Byte Integer" {
      n227 = Index Array(array=w628) -> (element=w632:string)  [unwired: 1 in]
      n228 = Index Array(array=w627) -> (element=w631:string)  [unwired: 1 in]
      n229 = Format Into String(format string="%s = (unsigned byte) %s;", w631, w632) -> (resulting string=w629:string)  [unwired: 2 in, 1 out]
    }
    frame "To Byte Integer" {
      n230 = Index Array(array=w634) -> (element=w638:string)  [unwired: 1 in]
      n231 = Index Array(array=w633) -> (element=w637:string)  [unwired: 1 in]
      n232 = Format Into String(format string="%s = (byte) %s;", w637, w638) -> (resulting string=w635:string)  [unwired: 2 in, 1 out]
    }
    frame "To Word Integer" {
      n233 = Index Array(array=w640) -> (element=w644:string)  [unwired: 1 in]
      n234 = Index Array(array=w639) -> (element=w643:string)  [unwired: 1 in]
      n235 = Format Into String(format string="%s = (short) %s;", w643, w644) -> (resulting string=w641:string)  [unwired: 2 in, 1 out]
    }
    frame "To Long Integer" {
      n236 = Index Array(array=w646) -> (element=w650:string)  [unwired: 1 in]
      n237 = Index Array(array=w645) -> (element=w649:string)  [unwired: 1 in]
      n238 = Format Into String(format string="%s = (long) %s;", w649, w650) -> (resulting string=w647:string)  [unwired: 2 in, 1 out]
    }
  }
  n239 = Set Variant Attribute(Variant=variant ("variant"), name="Replaced Code", value=w22) -> (Variant out=w10:variant)  [unwired: 1 in, 2 out]
  n240 = Set Variant Attribute(Variant=w10, name="Defines", value=w7) -> (Variant out=w9:variant)  [unwired: 1 in, 2 out]
  n241 = Set Variant Attribute(Variant=w9, name="Includes", value=w21) -> (Variant out=→"Output":variant)  [unwired: 1 in, 2 out]
  "error out" <- "error in (no error)"
